vi "tm488_attachbufferseq_wVision.vi"() -> ()   [LabVIEW 2021]
panel:
  out "Display":T1(plugin-control)
  out "DCAM Version":string
  out "Library Version":string
  out "Frames Per Second":dbl
  in  "Quit":bool
  out "Error Out":errorcluster {"code" format="%.0x"}
  # "This is an example of how to attach your own data buffers to the capture library."
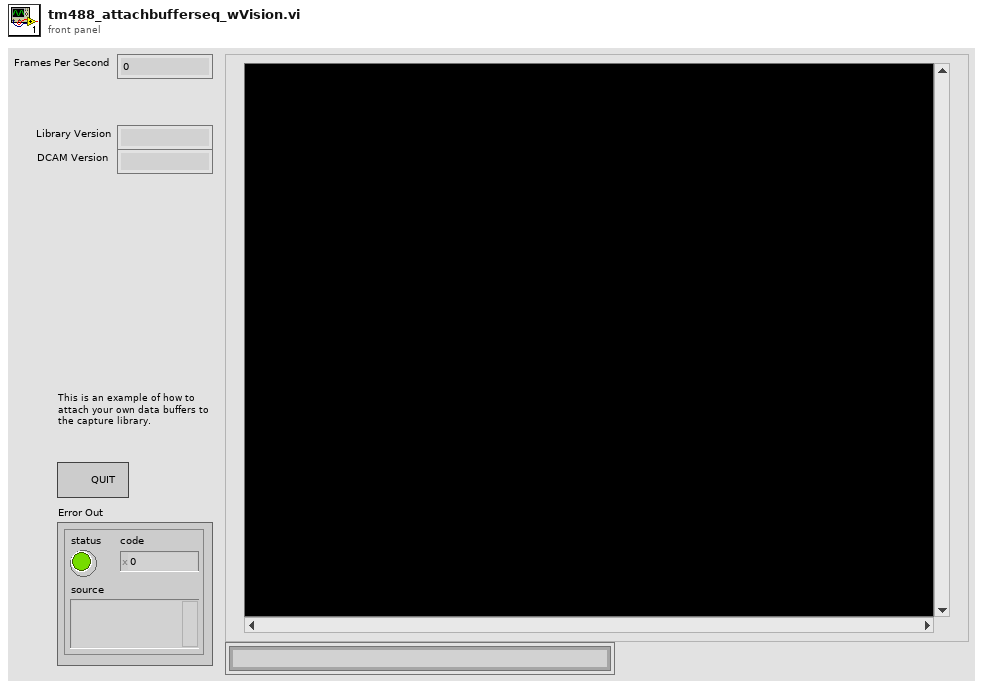
[diagram p1: front panel]
types:
  T1 = typedef "IMAQ Image.ctl" = refnum<image>
  T2 = cluster{"Capture Library":string, "DCAM-API":string}
  T3 = enum32{"Map Pixel Pointer", "Unmap Pixel Pointer", "Get Pixels Infos"}
  T4 = typedef "Image Type" = u32
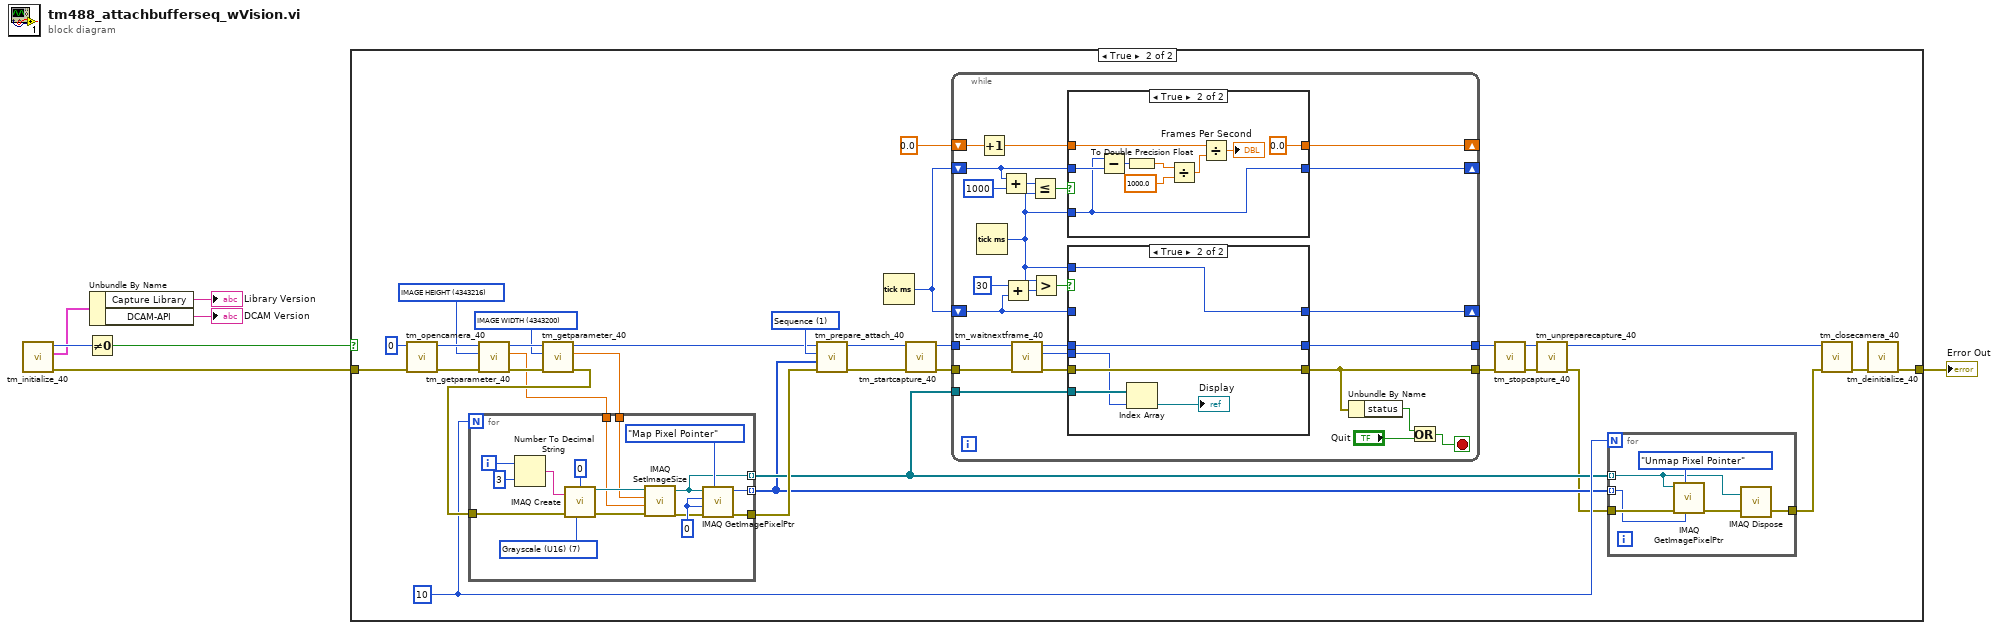
[diagram p0: block diagram]
diagram:
  n1 = call <userlib>:"tm_initialize_40.vi"() -> ("error out"=w4:errorcluster, "Version Info"=w3:T2, "Number Of Cameras"=w5:u32)  [unwired: 8 in, 1 out]
  n2 = Not Equal To 0?(x=w5) -> (x != 0?=w7:bool)
  n3 = Unbundle By Name(w3) -> ("Capture Library"=→"Library Version":string, "DCAM-API"=→"DCAM Version":string)
  n4 = case shown="True" w7 {
    tunnel: w4 -> [w8 w40]
    tunnel: [w8 w37] -> w6
    frame False {
    }
    frame True {
      w19 = u32 4343216 items=["SENSOR MODE"=4212128, "READOUT SPEED"=4211872, "READOUT DIRECTION"=4211904, "TRIGGER GLOBAL EXPOSURE"=2049680, "TRIGGER DELAY"=1066480, "INTERNAL TRIGGER HANDLING"=1066496, "SENSOR TEMPERATURE"=2115232, "SENSOR COOLER STATUS"=2115280, "EXPOSURE TIME"=2049184, "DEFECT CORRECT MODE"=4670368, "HOT PIXEL CORRECT LEVEL"=4670400, "BINNING"=4215968, "TIMING READOUT TIME"=4223904, "INTERNAL FRAME RATE"=4225952, "INTERNAL FRAME INTERVAL"=4225968, "INTERNAL LINE SPEED"=4226000, "INTERNAL LINE INTERVAL"=4226016, "IMAGE WIDTH"=4343200, "IMAGE HEIGHT"=4343216, "IMAGE ROWBYTES"=4343232, "IMAGE FRAMEBYTES"=4343248, "IMAGE PIXEL TYPE"=4343296, "NUMBER OF OUTPUT TRIGGER CONNECTOR"=1852320, "OUTPUT TRIGGER SOURCE[0]"=1852576, "OUTPUT TRIGGER SOURCE[1]"=1852832, "OUTPUT TRIGGER SOURCE[2]"=1853088, "OUTPUT TRIGGER POLARITY[0]"=1852592, "OUTPUT TRIGGER POLARITY[1]"=1852848, "OUTPUT TRIGGER POLARITY[2]"=1853104, "OUTPUT TRIGGER ACTIVE[0]"=1852608, "OUTPUT TRIGGER ACTIVE[1]"=1852864, "OUTPUT TRIGGER ACTIVE[2]"=1853120, "OUTPUT TRIGGER DELAY[0]"=1852624, "OUTPUT TRIGGER DELAY[1]"=1852880, "OUTPUT TRIGGER DELAY[2]"=1853136, "OUTPUT TRIGGER PERIOD[0]"=1852640, "OUTPUT TRIGGER PERIOD[1]"=1852896, "OUTPUT TRIGGER PERIOD[2]"=1853152, "OUTPUT TRIGGER KIND[0]"=1852656, "OUTPUT TRIGGER KIND[1]"=1852912, "OUTPUT TRIGGER KIND[2]"=1853168, "OUTPUT TRIGGER BASE SENSOR[0]"=1852672, "OUTPUT TRIGGER BASE SENSOR[1]"=1852928, "OUTPUT TRIGGER BASE SENSOR[2]"=1853184, "OUTPUT TRIGGER PRE HSYNC COUNT"=1852704] ("Parameter")
      w18 = u32 4343200 items=["SENSOR MODE"=4212128, "READOUT SPEED"=4211872, "READOUT DIRECTION"=4211904, "TRIGGER GLOBAL EXPOSURE"=2049680, "TRIGGER DELAY"=1066480, "INTERNAL TRIGGER HANDLING"=1066496, "SENSOR TEMPERATURE"=2115232, "SENSOR COOLER STATUS"=2115280, "EXPOSURE TIME"=2049184, "DEFECT CORRECT MODE"=4670368, "HOT PIXEL CORRECT LEVEL"=4670400, "BINNING"=4215968, "TIMING READOUT TIME"=4223904, "INTERNAL FRAME RATE"=4225952, "INTERNAL FRAME INTERVAL"=4225968, "INTERNAL LINE SPEED"=4226000, "INTERNAL LINE INTERVAL"=4226016, "IMAGE WIDTH"=4343200, "IMAGE HEIGHT"=4343216, "IMAGE ROWBYTES"=4343232, "IMAGE FRAMEBYTES"=4343248, "IMAGE PIXEL TYPE"=4343296, "NUMBER OF OUTPUT TRIGGER CONNECTOR"=1852320, "OUTPUT TRIGGER SOURCE[0]"=1852576, "OUTPUT TRIGGER SOURCE[1]"=1852832, "OUTPUT TRIGGER SOURCE[2]"=1853088, "OUTPUT TRIGGER POLARITY[0]"=1852592, "OUTPUT TRIGGER POLARITY[1]"=1852848, "OUTPUT TRIGGER POLARITY[2]"=1853104, "OUTPUT TRIGGER ACTIVE[0]"=1852608, "OUTPUT TRIGGER ACTIVE[1]"=1852864, "OUTPUT TRIGGER ACTIVE[2]"=1853120, "OUTPUT TRIGGER DELAY[0]"=1852624, "OUTPUT TRIGGER DELAY[1]"=1852880, "OUTPUT TRIGGER DELAY[2]"=1853136, "OUTPUT TRIGGER PERIOD[0]"=1852640, "OUTPUT TRIGGER PERIOD[1]"=1852896, "OUTPUT TRIGGER PERIOD[2]"=1853152, "OUTPUT TRIGGER KIND[0]"=1852656, "OUTPUT TRIGGER KIND[1]"=1852912, "OUTPUT TRIGGER KIND[2]"=1853168, "OUTPUT TRIGGER BASE SENSOR[0]"=1852672, "OUTPUT TRIGGER BASE SENSOR[1]"=1852928, "OUTPUT TRIGGER BASE SENSOR[2]"=1853184, "OUTPUT TRIGGER PRE HSYNC COUNT"=1852704] ("Parameter")
      w16 = 10
      w32 = 1 items=["Snap", "Sequence"] ("Capture mode")
      n5 = call <userlib>:"tm_opencamera_40.vi"("error in (no error)"=w40, "Camera Index"=u32 0) -> ("error out"=w25:errorcluster, "Handle out"=w24:u32)  [unwired: 7 in, 1 out]
      n6 = call <userlib>:"tm_getparameter_40.vi"("error in (no error)"=w25, "Parameter"=w19, "Handle in"=w24) -> ("error out"=w27:errorcluster, "Value out"=w17:dbl, "Handle out"=w26:u32)  [unwired: 6 in]
      n7 = call <userlib>:"tm_getparameter_40.vi"("error in (no error)"=w27, "Parameter"=w18, "Handle in"=w26) -> ("error out"=w23:errorcluster, "Value out"=w20:dbl, "Handle out"=w22:u32)  [unwired: 6 in]
      n8 = for {
        N: w16 -> [_]
        tunnel: [w51] -> w15 mode=indexing
        tunnel: [w56] -> w14 mode=indexing
        tunnel: w23 -> [w50]
        tunnel: [w49] -> w21
        tunnel: w20 -> [w48]
        tunnel: w17 -> [w47]
        i -> [w62]
        w53 = T4 7 items=["Grayscale (U8)", "Grayscale (I16)", "Grayscale (SGL)", "Complex (CSG)", "RGB (U32)", "HSL (U32)", "RGB (U64)", "Grayscale (U16)"] ("Image Type")
        w57 = 0 ("X Coordinate")
        n9 = Number To Decimal String(number=w62, width (-)=i16 3) -> (decimal integer string=w60:string)
        n10 = call "IMAQ Create"("Border Size"=0, "Image Name"=w60, "Image Type"=w53, "error in (no error)"=w50) -> ("New Image"=w55:T1, "error out"=w54:errorcluster)  [unwired: 1 in]
        n11 = call "IMAQ SetImageSize"("error in (no error)"=w54, "Y Resolution"=w47, "X Resolution"=w48, "Image"=w55) -> ("error out"=w52:errorcluster, "Image Out"=w51:T1)  [unwired: 1 in]
        n12 = call "IMAQ GetImagePixelPtr"("Function"=T3."Map Pixel Pointer", "error in (no error)"=w52, "Y Coordinate"=w57, "X Coordinate"=w57, "Image"=w51) -> ("error out"=w49:errorcluster, "Pixel Pointer out"=w56:u64)  [unwired: 1 in, 4 out]
      }
      n13 = call <userlib>:"tm_prepare_attach_40.vi"("error in (no error)"=w21, "buffers"=w14, "Capture mode"=w32, "Handle in"=w22) -> ("error out"=w30:errorcluster, "Handle out"=w31:u32)  [unwired: 6 in]
      n14 = Tick Count (ms)() -> (millisecond timer value=w28:u32)
      n15 = call <userlib>:"tm_startcapture_40.vi"("error in (no error)"=w30, "Handle in"=w31) -> ("error out"=w33:errorcluster, "Handle out"=w34:u32)  [unwired: 8 in]
      n16 = while {
        tunnel: [w66] -> w35
        tunnel: [w67] -> w36
        tunnel: w34 -> [w84]
        tunnel: w33 -> [w85]
        shift-right: [w82] -> _
        shift-left: w28 -> [w79]
        shift-right: [w83] -> _
        shift-left: 0.0 -> [w76]
        shift-right: [w65] -> _
        shift-left: w28 -> [w68]
        tunnel: w15 -> [w63]
        stop <- w64 stop-if-true
        n17 = Tick Count (ms)() -> (millisecond timer value=w69:u32)
        n18 = Increment(x=w76) -> (x+1=w77:dbl)
        n19 = Add(x=w79, y=u32 1000) -> (x+y=w81:u32)
        n20 = Add(x=u32 30, y=w68) -> (x+y=w71:u32)
        n21 = call <userlib>:"tm_waitnextframe_40.vi"("error in (no error)"=w85, "Handle in"=w84) -> ("error out"=w74:errorcluster, "Frame Index"=w73:i32, "Handle out"=w75:u32)  [unwired: 6 in, 1 out]
        n22 = Less Or Equal?(x=w81, y=w69) -> (x <= y?=w78:bool)
        n23 = Greater?(x=w69, y=w71) -> (0:w70:bool)
        n24 = case shown="True" w78 {
          tunnel: w79 -> [w98 w101]
          tunnel: [w98 w99] -> w82
          tunnel: w77 -> [w97 w105]
          tunnel: w69 -> [_ w99]
          tunnel: [w97 0.0] -> w83
          frame False {
          }
          frame True {
            n25 = Subtract(x=w99, y=w101) -> (x-y=w100:u32)
            n26 = To Double Precision Float(number=w100) -> (double precision float=w107:dbl)
            n27 = Divide(x=w107, y=1000.0) -> (x/y=w104:dbl)
            n28 = Divide(x=w105, y=w104) -> (x/y=→"Frames Per Second":dbl)
          }
        }
        n29 = case shown="True" w70 {
          tunnel: w75 -> [w90 w95]
          tunnel: w74 -> [w89 w94]
          tunnel: w73 -> [_ w92]
          tunnel: w68 -> [w88 _]
          tunnel: w69 -> [_ w96]
          tunnel: [w90 w95] -> w66
          tunnel: [w89 w94] -> w67
          tunnel: [w88 w96] -> w65
          tunnel: w63 -> [_ w93]
          frame False {
          }
          frame True {
            n30 = Index Array(array=w93, index=w92) -> (element=→"Display":T1)
          }
        }
        n31 = Unbundle By Name(w67) -> ("status"=w87:bool)
        n32 = Or(x=w87, y="Quit") -> (x .or. y?=w64:bool)
      }
      n33 = call <userlib>:"tm_stopcapture_40.vi"("error in (no error)"=w36, "Handle in"=w35) -> ("error out"=w13:errorcluster, "Handle out"=w12:u32)  [unwired: 8 in]
      n34 = call <userlib>:"tm_unpreparecapture_40.vi"("error in (no error)"=w13, "Handle in"=w12) -> ("error out"=w11:errorcluster, "Handle out"=w10:u32)  [unwired: 8 in]
      n35 = for {
        N: w16 -> [_]
        tunnel: w15 -> [w45] mode=indexing
        tunnel: w11 -> [w43]
        tunnel: [w42] -> w9
        tunnel: w14 -> [w41] mode=indexing
        n36 = call "IMAQ GetImagePixelPtr"("Pixel Pointer in"=w41, "Function"=T3."Unmap Pixel Pointer", "error in (no error)"=w43, "Image"=w45) -> ("error out"=w44:errorcluster)  [unwired: 2 in, 5 out]
        n37 = call "IMAQ Dispose"("Image"=w45, "error in (no error)"=w44) -> ("error out"=w42:errorcluster)  [unwired: 4 in]
      }
      n38 = call <userlib>:"tm_closecamera_40.vi"("error in (no error)"=w9, "Handle in"=w10) -> ("error out"=w38:errorcluster)  [unwired: 9 in]
      n39 = call <userlib>:"tm_deinitialize_40.vi"("error in (no error)"=w38) -> ("error out"=w37:errorcluster)  [unwired: 10 in]
    }
  }
  "Error Out" <- w6
